vi "Configure Limit Output.vi"(0 "VISA resource name":refnum<visa-resource-name>, 1 "Enable Limit Output Pulsing (False)":bool, 2 "Output Pulse Time (0.002 sec)":dbl=0.002, 5 "Enable Master Limit (False)":bool, 7 "Enable Limit Outputs (False)":bool, 9 "Logic Sense (0: Don't Configure)":u16(ring) items=["Don't Configure", "All Low", "All High"], 11 "error in (no error)":errorcluster) -> (4 "VISA resource name out":refnum<visa-resource-name>, 15 "error out":errorcluster)   [LabVIEW 2020, in "Keithley 27XX.lvlib"]
doc: "The digital I/O port (on the back of the instrument) has five digital outputs. Each digital output can be used as a sink to control devices (e.g., relays), or as a source to provide input to external logic (TTL or CMOS) circuitry. This VI will allow you to configure how this data will be output."
uses:
  Keithley 27XX.lvlib
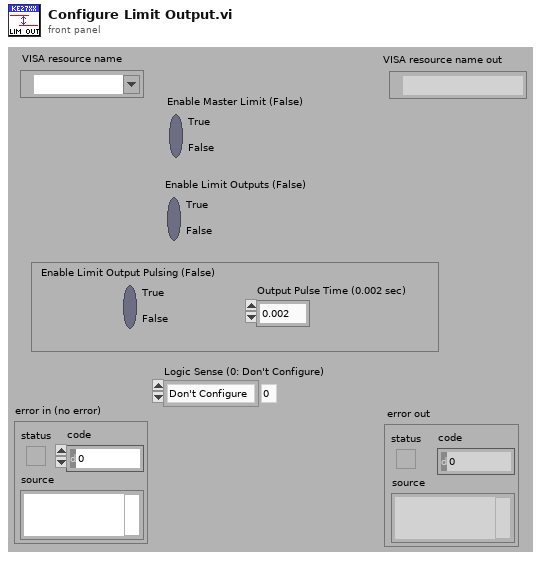
[diagram p1: front panel]
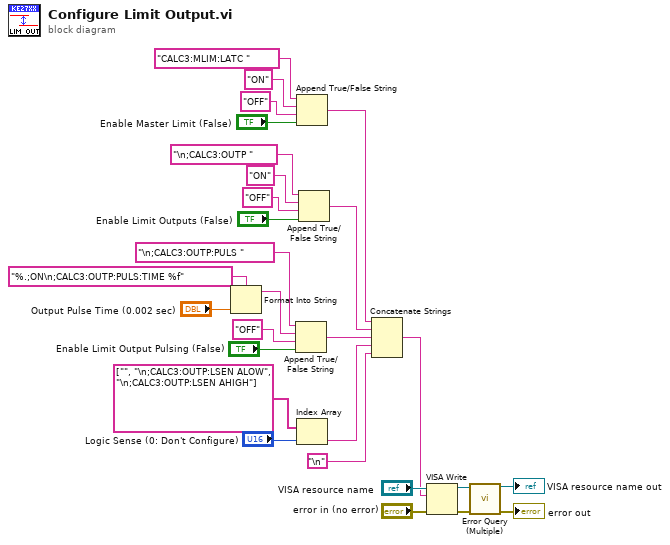
[diagram p0: block diagram]
diagram:
  n1 = Format Into String(format string="%.;ON\n;CALC3:OUTP:PULS:TIME %f", "Output Pulse Time (0.002 sec)") -> (resulting string=w27:string)  [unwired: 2 in, 1 out]
  n2 = Append True/False String(1:"Enable Limit Output Pulsing (False)", 2:"OFF" ("false string"), 3:w27, 4:"\n;CALC3:OUTP:PULS ") -> (0:w16:string)
  n3 = Append True/False String(1:"Enable Master Limit (False)", 2:"OFF", 3:"ON", 4:"CALC3:MLIM:LATC ") -> (0:w18:string)
  n4 = Index Array(array=string[] ["", "\n;CALC3:OUTP:LSEN ALOW", "\n;CALC3:OUTP:LSEN AHIGH"], index="Logic Sense (0: Don't Configure)") -> (element=w11:string)
  n5 = Append True/False String(1:"Enable Limit Outputs (False)", 2:"OFF", 3:"ON", 4:"\n;CALC3:OUTP ") -> (0:w17:string)
  n6 = Concatenate Strings(w18, w17, w16, w11, "\n") -> (w13:string)
  n7 = VISA Write(VISA resource name="VISA resource name", write buffer=w13, error in (no error)="error in (no error)") -> (VISA resource name out=w10:refnum<visa-resource-name>, error out=w9:errorcluster)  [unwired: 1 out]
  n8 = call "Error Query (Multiple).vi"("VISA resource name"=w10, "error in (no error)"=w9) -> ("VISA resource name out"=→"VISA resource name out":refnum<visa-resource-name>, "error out"=→"error out":errorcluster)  [unwired: 10 in, 2 out]
